vi "rqcBob Configure Pulse Train.vi"(8 "error in":errorcluster, 10 "train.configuration":T1={"period"=4000, "num of pulses"=1, "mode"=enum."train sequence.wait for trigger", "num of trains"=3000, "first pulse delay mode"=enum."every train", "first pulse delay"=55}, 11 "FPGA reference in":refnum<k20>) -> (0 "error out":errorcluster, 2 "SPD meas length":u32, 3 "FPGA reference out":refnum<k20>)   [LabVIEW 2019]
uses:
  FPGA/rqcBob/Custom Controls/Pulse Train/rqcBob Pulse Train Config.ctl
  FPGA/rqcBob/Custom Controls/Pulse Train/rqcBob Pulse Train.Generation Mode.ctl
  FPGA/rqcBob/Custom Controls/Pulse Train/rqcBob Pulse Train.First Pulse Delay Mode.ctl
  <vilib>/Utility/error.llb/Error Cluster From Error Code.vi
  <vilib>/rvi/errors/niLvFpgaAdjustHostInterfaceError.vi
  <vilib>/rvi/interface/nirviReadWriteControl/nirviReadWriteControl.xnode
  NiFpgaLv.dll
  <vilib>/rvi/interface/Simulation/niFpgaSimulationCallBeginRW.vi
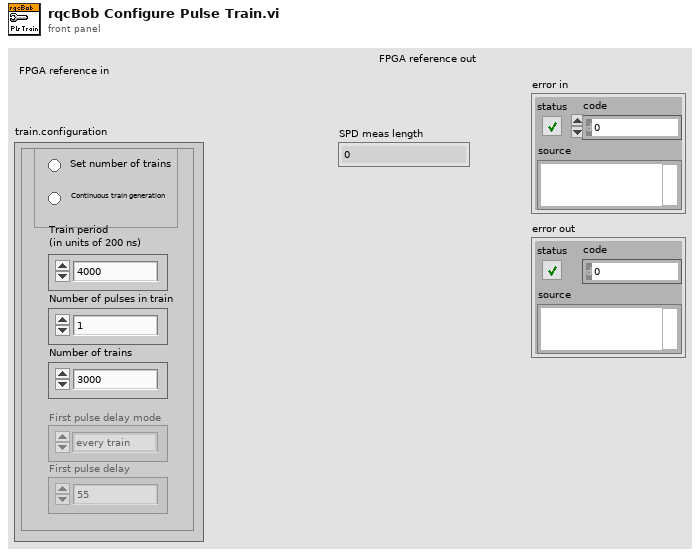
[diagram p1: front panel]
types:
  T1 = typedef "rqcBob Pulse Train Config.ctl" = cluster{"period":u16, "num of pulses":u16, "mode":T2, "num of trains":u16, "first pulse delay mode":T3, "first pulse delay":u16}
  T2 = typedef "rqcBob Pulse Train.Generation Mode.ctl" = enum32{"single train", "train sequence.single", "train sequence.wait for trigger", "continuous"}
  T3 = typedef "rqcBob Pulse Train.First Pulse Delay Mode.ctl" = enum8{"none", "every train", "first train"}
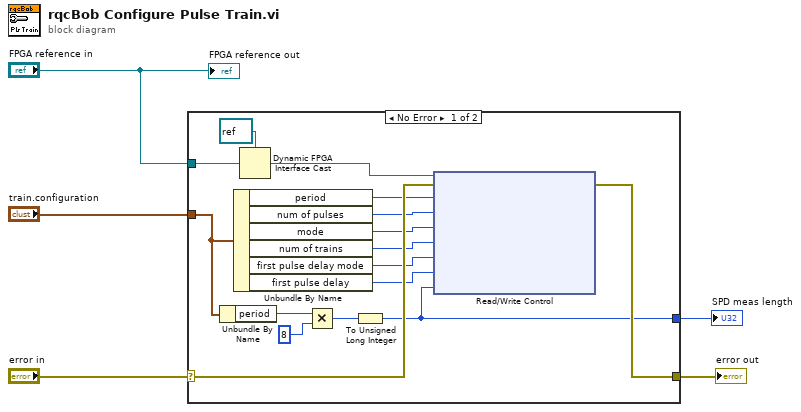
[diagram p0: block diagram]
diagram:
  n1 = case shown="No Error" "error in" {
    selector: "error in" -> [w21 w22]
    tunnel: [w20 w22] -> w3
    tunnel: "FPGA reference in" -> [w18 _]
    tunnel: "train.configuration" -> [w13 _]
    tunnel: [w12 _] -> w1
    frame No Error {
      n2 = Unbundle By Name(w13) -> ("period"=w16:u16)
      n3 = Unbundle By Name(w13) -> ("period"=w11:u16, "num of pulses"=w10:u16, "mode"=w9:T2, "num of trains"=w8:u16, "first pulse delay mode"=w7:T3, "first pulse delay"=w6:u16)
      n4 = Dynamic FPGA Interface Cast(Session In=refnum<k20> refnum ("FPGA Interface"), Type=w18) -> (Session Out=w17:refnum<k20>)
      n5 = Multiply(x=w16, y=u16 8) -> (x*y=w14:u16)
      n6 = To Unsigned Long Integer(number=w14) -> (unsigned 32bit integer=w12:u32)
      n7 = xnode "Read/Write Control"("FPGA VI Reference In"=w17, "error in"=w21, "train.period"=w11, "train.num of pulses"=w10, "train.mode"=w9, "train.num of trains"=w8, "train.first pulse delay mode"=w7, "train.first pulse delay"=w6, "PD.max meas length"=w12) -> ("error out"=w20:errorcluster)  [unwired: 1 out]
    }
    frame Error {
    }
  }
  "error out" <- w3
  "SPD meas length" <- w1
  "FPGA reference out" <- "FPGA reference in"
